vi "WF Gap Creator.vi"(8 "error in":errorcluster, 10 "Character Gap":u8, 11 "Unit Speed":dbl) -> (0 "error out":errorcluster, 3 "waveform out":waveform(dbl))   [LabVIEW 2026]
doc: "Create the gaps between chars and words."
uses:
  <vilib>/measure/NI_MABase.lvlib
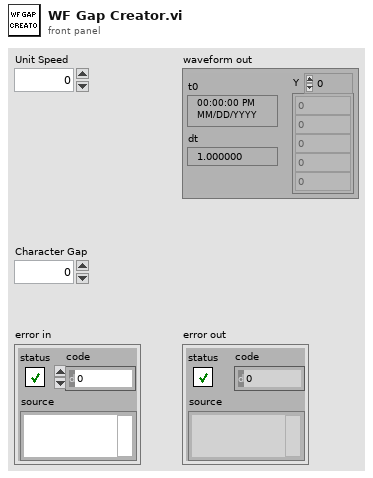
[diagram p1: front panel]
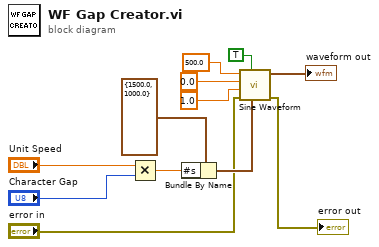
[diagram p0: block diagram]
diagram:
  n1 = Multiply(x="Unit Speed", y="Character Gap") -> (x*y=w11:dbl)
  n2 = Bundle By Name(cluster=cluster{"Fs":dbl, "#s":dbl} {"Fs"=1500.0, "#s"=1000.0} ("sampling info"), "#s"=w11) -> (w8:cluster{"Fs":dbl, "#s":dbl})
  n3 = call <vilib>:"Sine Waveform.vi"("sampling info"=w8, "reset signal"=TRUE, "error in (no error)"="error in", "phase"=1.0, "amplitude"=0.0, "frequency"=500.0) -> ("error out"=→"error out":errorcluster, "signal out"=→"waveform out":waveform(dbl))  [unwired: 4 in]
